vi "Read all Controls.vi"(8 "error in (no error)":errorcluster, 11 "Sim User Console Actor in":refnum<class "Sim User Console Actor.lvclass">) -> (0 "error out":errorcluster, 3 "Sim User Console Actor out":refnum<class "Sim User Console Actor.lvclass">)   [LabVIEW 2019, in "Simulated User Console Actor.lvlib" / "Sim User Console Actor.lvclass"]
uses:
  Sim User Console Actor.lvclass
  Elevator Controller/Elevator Controller Actor Messages/No request remaining Msg/No request remaining Msg.lvclass
  <vilib>/ActorFramework/Actor/Actor.lvclass
  C:/Workspace/CLA/Elevator AF 2nd/User Console Actor/User Console Actor/User Console Actor.lvclass
  C:/Program Files (x86)/National Instruments/LabVIEW 2019/vi.lib/ActorFramework/Actor/Actor.lvclass
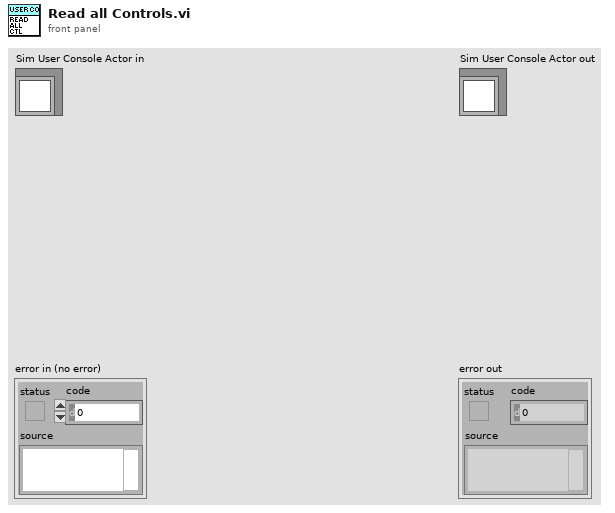
[diagram p1: front panel]
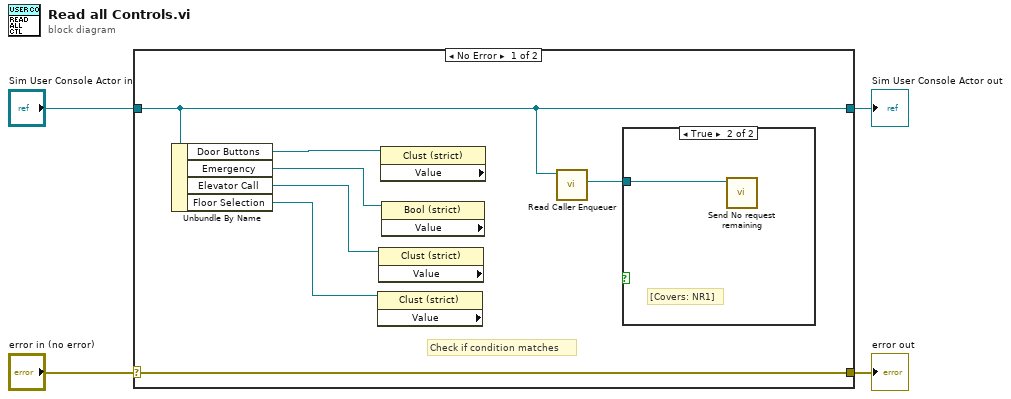
[diagram p0: block diagram]
diagram:
  n1 = case shown="No Error" "error in (no error)" {
    selector: "error in (no error)" -> [w11 w14]
    tunnel: [w11 w14] -> w3
    tunnel: [w6 w13] -> w1
    tunnel: "Sim User Console Actor in" -> [w6 w13]
    frame No Error {
      # "Check if condition matches"
      n2 = Unbundle By Name(w6) -> ("Door Buttons"=w10:refnum<vi>, "Emergency"=w9:refnum<vi>, "Elevator Call"=w8:refnum<vi>, "Floor Selection"=w7:refnum<vi>)
      n3 = property class="Clust (strict)" props=["Value"](reference=w7) -> ()  [unwired: 1 in, 3 out]
      n4 = property class="Clust (strict)" props=["Value"](reference=w8) -> ()  [unwired: 1 in, 3 out]
      n5 = property class="Clust (strict)" props=["Value"](reference=w10) -> ()  [unwired: 1 in, 3 out]
      n6 = property class="Bool (strict)" props=["Value"](reference=w9) -> ()  [unwired: 1 in, 3 out]
      n7 = call <vilib>:"Read Caller Enqueuer.vi"("Actor"=w6) -> ("Caller Enqueuer"=w5:refnum<class "Message Enqueuer.lvclass">)  [unwired: 10 in]
      n8 = case shown="True" {
        selector: _ -> [_ _]
        tunnel: w5 -> [_ w12]
        frame False {
        }
        frame True {
          # "[Covers: NR1]"
          n9 = call "Send No request remaining.vi"("Message Enqueuer"=w12) -> ()  [unwired: 9 in, 2 out]
        }
      }
    }
    frame Error {
    }
  }
  "error out" <- w3
  "Sim User Console Actor out" <- w1
